vi "DataGraph_MouseBoundaryCalc.vi"(1 "Minimum":dbl, 2 "Maximum":dbl, 3 "Value in":dbl) -> (0 "Value out":dbl)   [LabVIEW 2018, in "DataGraphXControl.xctl"]
uses:
  DataGraphXControl.xctl
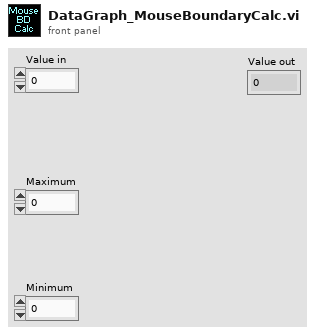
[diagram p1: front panel]
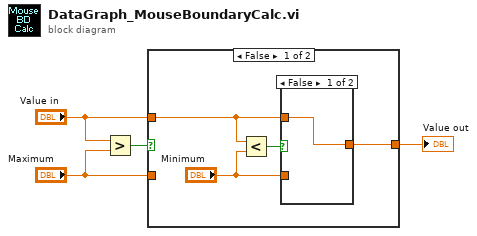
[diagram p0: block diagram]
diagram:
  n1 = Greater?(x="Value in", y="Maximum") -> (0:w4:bool)
  n2 = case shown="False" w4 {
    tunnel: "Maximum" -> [_ w11]
    tunnel: [w5 w11] -> w1
    tunnel: "Value in" -> [w7 _]
    frame False {
      n3 = Less?(x=w7, y="Minimum") -> (x < y?=w6:bool)
      n4 = case shown="False" w6 {
        tunnel: "Minimum" -> [_ w10]
        tunnel: w7 -> [w9 _]
        tunnel: [w9 w10] -> w5
        frame False {
        }
        frame True {
        }
      }
    }
    frame True {
    }
  }
  "Value out" <- w1
